vi "update globals from exec.vi"(11 "PID exp exec":T2, 12 "exec.T mode":T1) -> (8 "Total elapsed time (s)":dbl=30.0, 15 "PID exp exec out":T2)   [LabVIEW 2019]
doc: "This subVI updates the bug global variables from the executive thread.\n\nPaul K Dixon\nP3600\nCSUSB Physics"
uses:
  typedefs/temp cont cluster.ctl
  typedefs/temp exec cluster.ctl
  typedefs/temp mode enum.ctl
  typedefs/temp indicator.ctl
  typedefs/temp cont utility.ctl
  typedefs/PID exec cluster.ctl
  globals/Bug man temp globals.vi
panel:
  out "T cont out":T3 {"utility"."therm volt" format="%_6g"; "T status"."Temp" format="%_6g"}
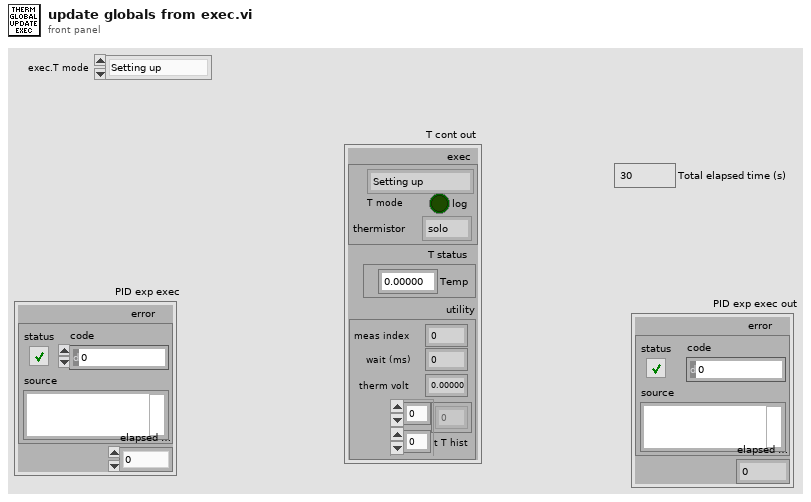
[diagram p1: front panel]
types:
  T1 = typedef "temp mode enum.ctl" = enum16{"Setting up", "Listening to exec", "Exit"}
  T2 = typedef "PID exec cluster.ctl" = cluster{"error":errorcluster, "elapsed time (s)":dbl}
  T3 = typedef "temp cont cluster.ctl" = cluster{"exec":T4, "T status":T5, "utility":T6}
  T4 = typedef "temp exec cluster.ctl" = cluster{"T mode":T1, "log":bool, "thermistor":enum16{"solo", "bug"}}
  T5 = typedef "temp indicator.ctl" = cluster{"Temp":dbl}
  T6 = typedef "temp cont utility.ctl" = cluster{"meas index":i32, "wait (ms)":i32, "therm volt":dbl, "t T hist":dbl[][]}
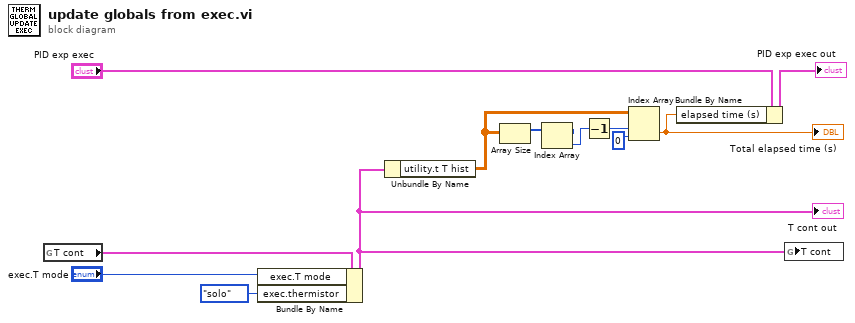
[diagram p0: block diagram]
diagram:
  n1 = global read "Bug man temp globals.vi" "T cont"() -> (w11:T3)
  n2 = Bundle By Name(cluster=w11, "exec.T mode"="exec.T mode", "exec.thermistor"=enum16{"solo", "bug"}."solo") -> (w10:T3)
  "T cont out" <- w10
  n3 = Unbundle By Name(w10) -> ("utility.t T hist"=w8:dbl[][])
  n4 = Array Size(array=w8) -> (size(s)=w5:i32[])
  n5 = Index Array(array=w5) -> (element=w4:i32)  [unwired: 1 in]
  n6 = Decrement(x=w4) -> (x-1=w6:i32)
  n7 = Index Array(array=w8, index (row)=w6, index (col)=0 ("disabled index (col)")) -> (element=w2:dbl)
  "Total elapsed time (s)" <- w2
  n8 = Bundle By Name(cluster="PID exp exec", "elapsed time (s)"=w2) -> (→"PID exp exec out":T2)
  n9 = global write "Bug man temp globals.vi" "T cont"(w10) -> ()
